vi "Split Array.vi"(9 "Number of Segments":i32, 11 "Array":u32[][](array[numeric])) -> (2 "Offsets":T1[](array[typedef]), 3 "Split Array":u32[][][](array[numeric]))   [LabVIEW 2018]
uses:
  Coordinate STYP.ctl
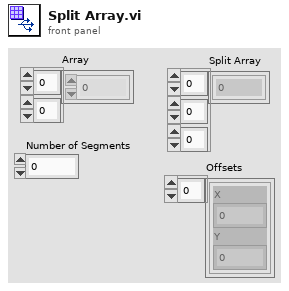
[diagram p1: front panel]
types:
  T1 = typedef "Coordinate STYP.ctl" = cluster{"X":i32, "Y":i32}
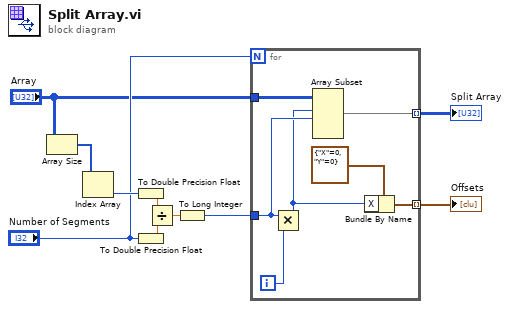
[diagram p0: block diagram]
diagram:
  n1 = Array Size(array="Array") -> (size(s)=w10:i32[])
  n2 = Index Array(array=w10) -> (element=w8:i32)  [unwired: 1 in]
  n3 = To Double Precision Float(number=w8) -> (double precision float=w9:dbl)
  n4 = To Double Precision Float(number="Number of Segments") -> (double precision float=w7:dbl)
  n5 = Divide(x=w9, y=w7) -> (x/y=w6:dbl)
  n6 = To Long Integer(number=w6) -> (32bit integer=w4:i32)
  n7 = for {
    N: "Number of Segments" -> [_]
    tunnel: w4 -> [w15]
    tunnel: "Array" -> [w17]
    tunnel: [w14] -> w2 mode=indexing
    tunnel: [w11] -> w1 mode=indexing
    i -> [w16]
    n8 = Multiply(x=w15, y=w16) -> (x*y=w12:i32)
    n9 = Array Subset(array=w17, index (row)=w12, length (row)=w15) -> (w14:u32[][])  [unwired: 2 in]
    n10 = Bundle By Name(cluster=T1 {"X"=0, "Y"=0} ("Coordinate"), "X"=w12) -> (w11:T1)
  }
  "Split Array" <- w2
  "Offsets" <- w1
